vi "LEBITplc.2dArrayToFile.vi"(2 "file path (dialog if empty)":path, 3 "Array":string[][](array[string])) -> ()   [LabVIEW 2014, in "LEBITplc.lvlib"]
uses:
  LEBITplc.lvlib
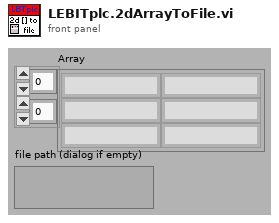
[diagram p1: front panel]
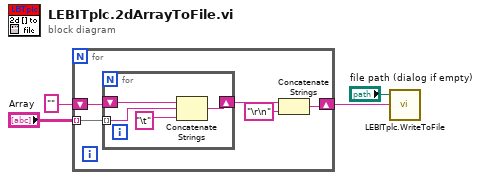
[diagram p0: block diagram]
diagram:
  n1 = for "For all Elements" {
    tunnel: "Array" -> [w9] mode=indexing
    shift-right: [w5] -> w2
    shift-left: "" -> [w8]
    n2 = for {
      tunnel: w9 -> [w12] mode=indexing
      shift-right: [w10] -> w7
      shift-left: w8 -> [w13]
      n3 = Concatenate Strings(w13, w12, "\t") -> (w10:string)
    }
    n4 = Concatenate Strings(w7, "\r\n") -> (w5:string)
  }
  n5 = call "LEBITplc.WriteToFile.vi"("character string"=w2, "file path (dialog if empty)"="file path (dialog if empty)") -> ()  [unwired: 3 in, 1 out]
